vi "Check Empty JSON String.vi"(11 "JSON":string) -> (3 "JSON":string)   [LabVIEW 2020, in "wamplv.lvlib" / "WAMP Client.lvclass"]
uses:
  <userlib>/wamplv/WAMP Client/WAMP Client.lvclass
  <userlib>/wamplv/WAMP Client/WAMP Client.lvclass/WAMP Client.ctl
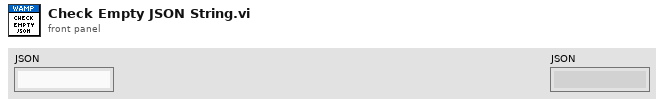
[diagram p1: front panel]
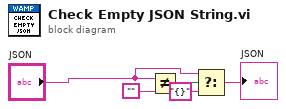
[diagram p0: block diagram]
diagram:
  n1 = Not Equal?(x="JSON", y="") -> (x != y?=w4:bool)
  n2 = Select(t="JSON", s=w4, f="{}") -> (s? t:f=→"JSON":string)
